vi "20_Basics of Cluster.vi"() -> ()   [LabVIEW 2018]
panel:
  out "Waveform Graph":dbl[](graph)
  out "Output String Cluster":cluster{"String":string, "String 2":string}
  out "x+y":cluster{"Array":dbl[], "Numeric":dbl}
  in  "Cluster 2":T1
  in  "Cluster":T1
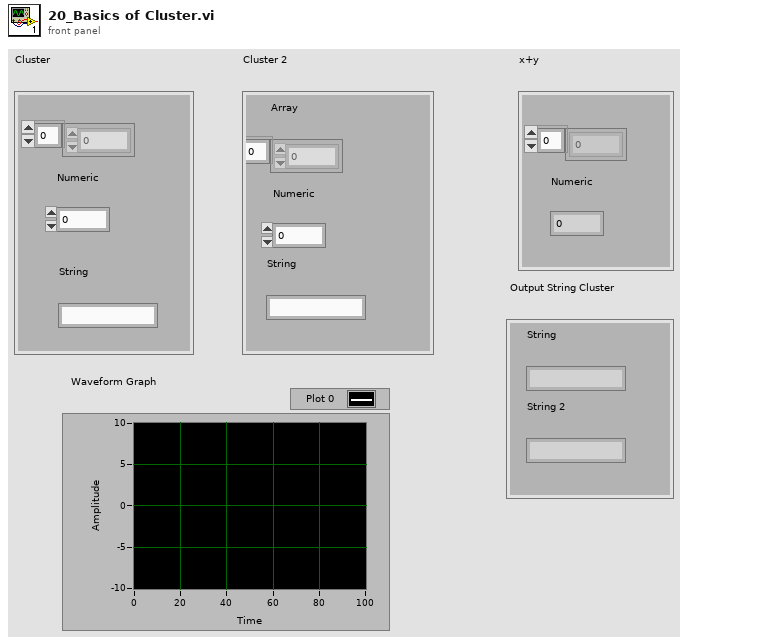
[diagram p1: front panel]
types:
  T1 = cluster{"Array":dbl[], "Numeric":dbl, "String":string}
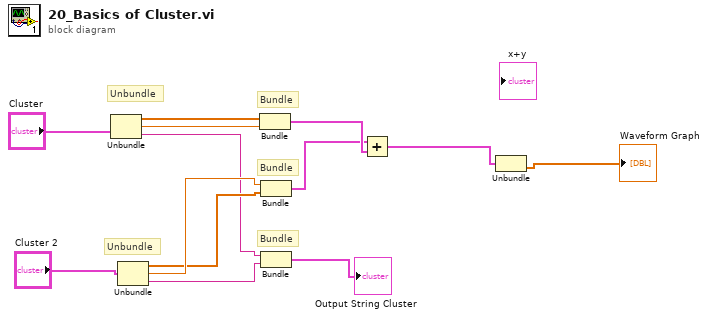
[diagram p0: block diagram]
diagram:
  # "Bundle"
  # "Bundle"
  # "Bundle"
  # "Unbundle"
  # "Unbundle"
  n1 = Unbundle("Cluster") -> ("Array"=w10:dbl[], "Numeric"=w11:dbl, "String"=w7:string)
  n2 = Unbundle("Cluster 2") -> ("Array"=w8:dbl[], "Numeric"=w9:dbl, "String"=w6:string)
  n3 = Bundle("Numeric"=w11, "Array"=w10) -> (w3:cluster{"Numeric":dbl, "Array":dbl[]})  [unwired: 1 in]
  n4 = Bundle("Numeric"=w9, "Array"=w8) -> (w2:cluster{"Numeric":dbl, "Array":dbl[]})  [unwired: 1 in]
  n5 = Bundle("String"=w7, "String"=w6) -> (→"Output String Cluster":cluster{"String":string, "String":string})  [unwired: 1 in]
  n6 = Add(x=w2, y=w3) -> (x+y=w1:cluster{"Numeric":dbl, "Array":dbl[]})
  n7 = Unbundle(w1) -> ("Array"=→"Waveform Graph":dbl[])  [unwired: 1 out]
